vi "Get Properties.vi"(8 "error in":errorcluster, 9 "Scope (0:All)":enum16{"All", "Dynamic"}(ring), 10 "AppInst":refnum<vi>, 11 "VI Name":string caption="VI Name (\"\")") -> (0 "error out":errorcluster, 1 "Column Data Type":enum16{"String", "Numeric"}[](array[ring]), 2 "Column Labels":string[](array[string])=["VI Name", "State", "Reentrant", "Reentrancy Type", "FP Behavior", "Code Size", "Data Size", "VI Path"], 3 "Full Name Out":string, 4 "VI Properties (All)":string[](array[string]), 5 "File Name Out":string, 6 "VI Properties (Dyn)":string[](array[string]))   [LabVIEW 2013]
doc: "Gets the properties at run time of each VI in memory. Set Scope=All to get all properties, set Scope=Dynamic to get only the properties that might change while executing. The later mode will be faster."
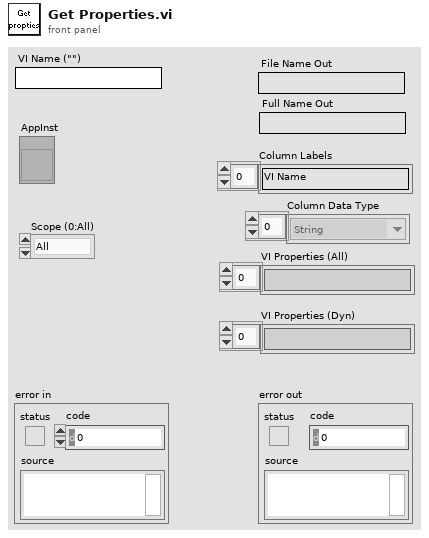
[diagram p1: front panel]
types:
  T1 = enum32{"Bad", "Idle", "Run top level", "Running"}
  T2 = enum16{"Share clones between instances", "Preallocate clone for each instance"}
  T3 = enum32{"Invalid", "Default", "Floating", "Floating/Auto-Hide", "Modal"}
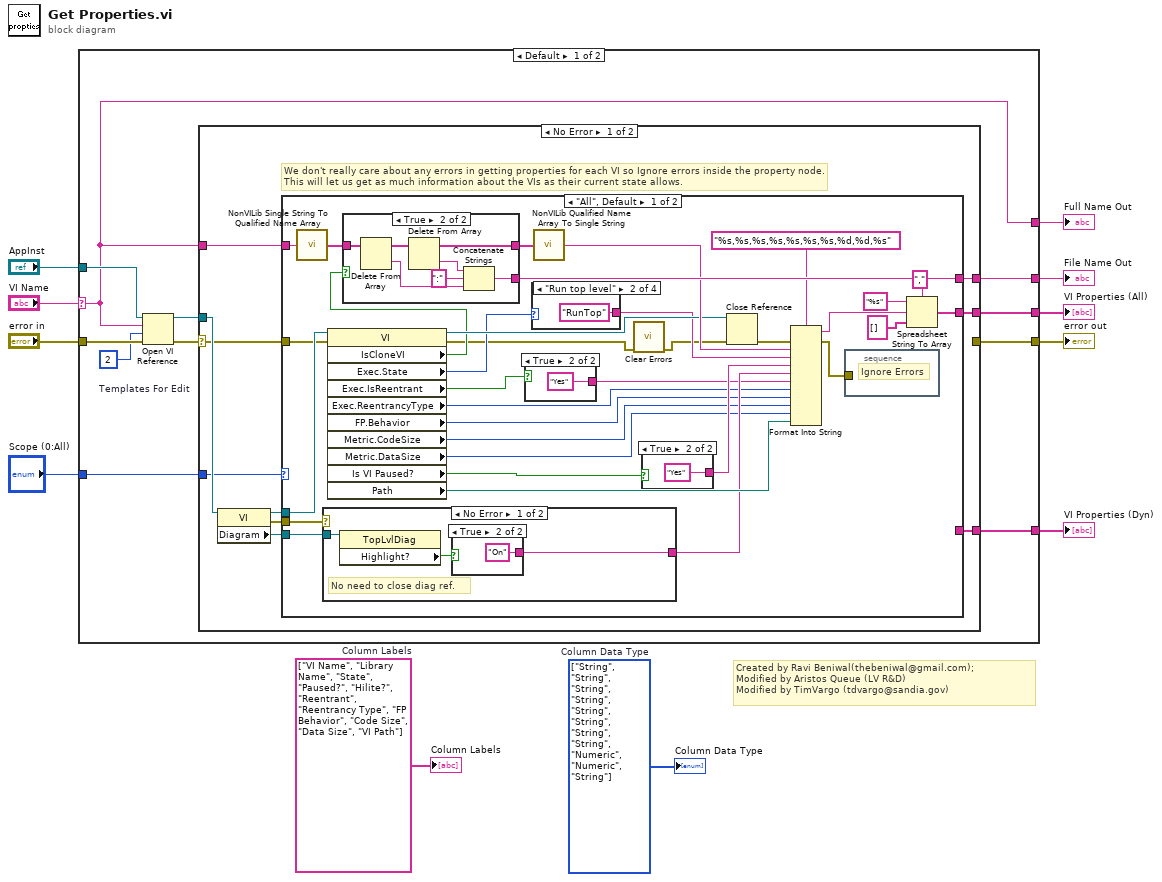
[diagram p0: block diagram]
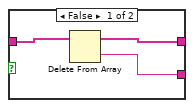
[diagram p2: hidden frame]
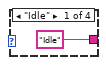
[diagram p4: hidden frame]
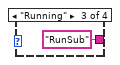
[diagram p5: hidden frame]
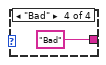
[diagram p6: hidden frame]
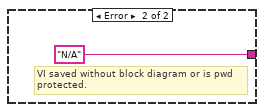
[diagram p8: hidden frame]
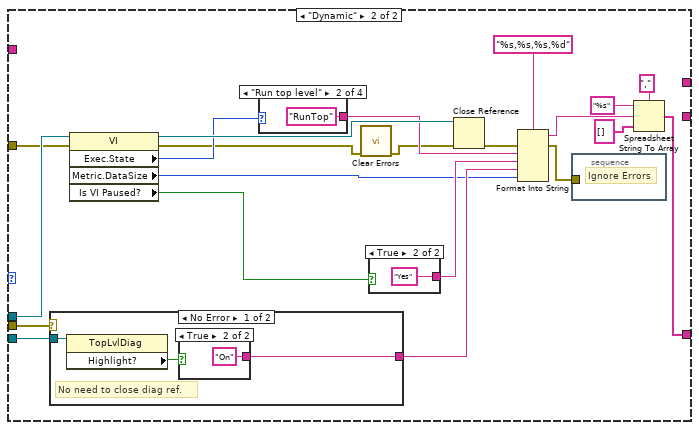
[diagram p10: hidden frame]
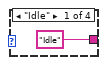
[diagram p11: hidden frame]
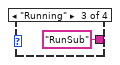
[diagram p12: hidden frame]
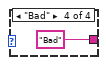
[diagram p13: hidden frame]
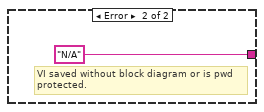
[diagram p15: hidden frame]
diagram:
  w7 = enum16{"String", "Numeric"}[] [enum."String", enum."String", enum."String", enum."String", enum."String", enum."String", enum."String", enum."String", enum."Numeric", enum."Numeric", enum."String"] items=["String", "Numeric"]  # Column Data Type
  w10 = string[] ["VI Name", "Library Name", "State", "Paused?", "Hilite?", "Reentrant", "Reentrancy Type", "FP Behavior", "Code Size", "Data Size", "VI Path"]  # Column Labels
  # "Created by Ravi Beniwal(thebeniwal@gmail.com);\nModified by Aristos Queue (LV R&D)\nModified by TimVargo (tdvargo@sandia.gov)"
  n1 = case shown="Default" "VI Name" {
    selector: "VI Name" -> [w16 w120]
    tunnel: [w22 _] -> w11
    tunnel: "error in" -> [w21 w119]
    tunnel: [w16 w120] -> w8
    tunnel: [w18 _] -> w6
    tunnel: "AppInst" -> [w17 _]
    tunnel: [w14 w119] -> w3
    tunnel: "Scope (0:All)" -> [w13 _]
    tunnel: [w12 _] -> w1
    frame Default {
      w19 = 2  # Templates For Edit
      n2 = Open VI Reference(application reference (local)=w17, vi path=w16, options=w19, error in (no error)=w21) -> (vi reference=w20:refnum<vi>, error out=w15:errorcluster)  [unwired: 2 out]
      n3 = case shown="No Error" w15 {
        selector: w15 -> [w25 w118]
        tunnel: [w32 _] -> w22
        tunnel: w20 -> [w31 _]
        tunnel: [w30 _] -> w18
        tunnel: w16 -> [w29 _]
        tunnel: [_ w118] -> w14
        tunnel: w13 -> [w24 _]
        tunnel: [w23 _] -> w12
        frame No Error {
          # "We don't really care about any errors in getting properties for each VI so Ignore errors inside the property node.\nThis will let us get as much information about the VIs as their current state allows."
          n4 = property class="VI"(reference=w31) -> (reference out=w27:refnum<vi>, error out=w28:errorcluster, "Diagram"=w26:refnum<vi>)  [unwired: 1 in]
          n5 = case shown="\"All\", Default" w24 {
            tunnel: [w65 _] -> w32
            tunnel: [w64 _] -> w30
            tunnel: w29 -> [w63 _]
            tunnel: w28 -> [w50 w99]
            tunnel: w27 -> [w49 w98]
            tunnel: w26 -> [w48 w97]
            tunnel: w25 -> [w33 w88]
            tunnel: [_ w87] -> w23
            frame "All", Default {
              n6 = call "NonVILib Single String To Qualified Name Array.vi"("Fully Qualified String"=w63) -> ("Fully Qualified Array"=w62:string[])
              n7 = case shown="No Error" w50 {
                tunnel: [w81 "N/A"] -> w44
                tunnel: w48 -> [w83 _]
                frame No Error {
                  # "No need to close diag ref."
                  n8 = property class="TopLvlDiag"(reference=w83) -> ("Highlight?"=w82:bool)  [unwired: 1 in, 2 out]
                  n9 = case shown="True" w82 {
                    tunnel: [_ "On"] -> w81
                    frame False {
                    }
                    frame True {
                    }
                  }
                }
                frame Error {
                  # "VI saved without block diagram or is pwd protected."
                }
              }
              n10 = property class="VI"(reference=w49, error in=w33) -> (reference out=w59:refnum<vi>, error out=w34:errorcluster, "IsCloneVI"=w36:bool, "Exec.State"=w47:T1, "Exec.IsReentrant"=w39:bool, "Exec.ReentrancyType"=w40:T2, "FP.Behavior"=w41:T3, "Metric.CodeSize"=w42:u32, "Metric.DataSize"=w43:u32, "Is VI Paused?"=w51:bool, "Path"=w52:path)
              n11 = case shown="True" w36 {
                tunnel: w62 -> [w68 w75]
                tunnel: [w67 w69] -> w64
                tunnel: [w66 w73] -> w61
                frame False {
                  n12 = Delete From Array(array=w68) -> (deleted portion=w67:string, array with subset deleted=w66:string[])  [unwired: 2 in]
                }
                frame True {
                  n13 = Delete From Array(array=w75) -> (deleted portion=w71:string, array with subset deleted=w74:string[])  [unwired: 2 in]
                  n14 = Delete From Array(array=w74) -> (deleted portion=w72:string, array with subset deleted=w73:string[])  [unwired: 2 in]
                  n15 = Concatenate Strings(w72, ":" ("element"), w71) -> (w69:string)
                }
              }
              n16 = case shown="True" w39 {
                tunnel: [_ "Yes"] -> w38
                frame False {
                }
                frame True {
                }
              }
              n17 = case shown="\"Run top level\"" w47 {
                tunnel: ["Idle" "RunTop" "RunSub" "Bad"] -> w46
                frame "Idle" {
                }
                frame "Run top level" {
                }
                frame "Running" {
                }
                frame "Bad" {
                }
              }
              n18 = call "NonVILib Qualified Name Array To Single String.vi"("Fully Qualified Array"=w61) -> ("Fully Qualified String"=w60:string)
              n19 = call <vilib>:"Clear Errors.vi"("error in (no error)"=w34) -> ("error out"=w35:errorcluster)  [unwired: 6 in]
              n20 = case shown="True" w51 {
                tunnel: [_ "Yes"] -> w45
                frame False {
                }
                frame True {
                }
              }
              n21 = Close Reference(reference=w59, error in (no error)=w35) -> (error out=w56:errorcluster)
              n22 = Format Into String(format string="%s,%s,%s,%s,%s,%s,%s,%d,%d,%s", error in=w56, w60, w46, w45, w44, w38, w40, w41, w42, w43, w52) -> (resulting string=w53:string, error out=w37:errorcluster)  [unwired: 1 in]
              n23 = stacked-sequence {
                tunnel: w37 -> [_]
                frame #0 {
                  # "Ignore Errors"
                }
              }
              n24 = Spreadsheet String To Array(delimiter (Tab)=",", format string="%s", spreadsheet string=w53, array type (2D Dbl)=string[] [] ("appended array")) -> (array=w65:string[])
            }
            frame "Dynamic" {
              n25 = case shown="No Error" w99 {
                tunnel: [w112 "N/A"] -> w93
                tunnel: w97 -> [w114 _]
                frame No Error {
                  # "No need to close diag ref."
                  n26 = property class="TopLvlDiag"(reference=w114) -> ("Highlight?"=w113:bool)  [unwired: 1 in, 2 out]
                  n27 = case shown="True" w113 {
                    tunnel: [_ "On"] -> w112
                    frame False {
                    }
                    frame True {
                    }
                  }
                }
                frame Error {
                  # "VI saved without block diagram or is pwd protected."
                }
              }
              n28 = property class="VI"(reference=w98, error in=w88) -> (reference out=w107:refnum<vi>, error out=w89:errorcluster, "Exec.State"=w96:T1, "Metric.DataSize"=w92:u32, "Is VI Paused?"=w100:bool)
              n29 = case shown="\"Run top level\"" w96 {
                tunnel: ["Idle" "RunTop" "RunSub" "Bad"] -> w95
                frame "Idle" {
                }
                frame "Run top level" {
                }
                frame "Running" {
                }
                frame "Bad" {
                }
              }
              n30 = call <vilib>:"Clear Errors.vi"("error in (no error)"=w89) -> ("error out"=w90:errorcluster)  [unwired: 6 in]
              n31 = case shown="True" w100 {
                tunnel: [_ "Yes"] -> w94
                frame False {
                }
                frame True {
                }
              }
              n32 = Close Reference(reference=w107, error in (no error)=w90) -> (error out=w104:errorcluster)
              n33 = Format Into String(format string="%s,%s,%s,%d", error in=w104, w95, w94, w93, w92) -> (resulting string=w101:string, error out=w91:errorcluster)  [unwired: 1 in]
              n34 = stacked-sequence {
                tunnel: w91 -> [_]
                frame #0 {
                  # "Ignore Errors"
                }
              }
              n35 = Spreadsheet String To Array(delimiter (Tab)=",", format string="%s", spreadsheet string=w101, array type (2D Dbl)=string[] [] ("appended array")) -> (array=w87:string[])
            }
          }
        }
        frame Error {
          # "Item is no longer in memory! Pass an error so it can be removed from the Task Manager."
        }
      }
    }
    frame "" {
      # "Addin this blank case let's us use this VI for getting the Col headers. \nIt is just easier to manage the column headers and getting their values in one VI."
    }
  }
  "error out" <- w3
  "VI Properties (All)" <- w11
  "Full Name Out" <- w8
  "File Name Out" <- w6
  "VI Properties (Dyn)" <- w1
  "Column Labels" <- w10
  "Column Data Type" <- w7
